vi "Change Behavior.vi"(8 "error in (no error)":errorcluster, 10 "New UI Actor":refnum<class "Flex UI (Actor).lvclass">, 11 "Flex UI (Actor) in":refnum<class "Flex UI (Actor).lvclass">) -> (0 "error out":errorcluster, 3 "Flex UI (Actor) out":refnum<class "Flex UI (Actor).lvclass">)   [LabVIEW 2014, in "Flex UI (Parent Actor).lvlib" / "Flex UI (Actor).lvclass"]
uses:
  Flex UI (Actor).lvclass
  <vilib>/East West Architects/Flex UI/Flex UI (Parent)/Flex UI.lvclass
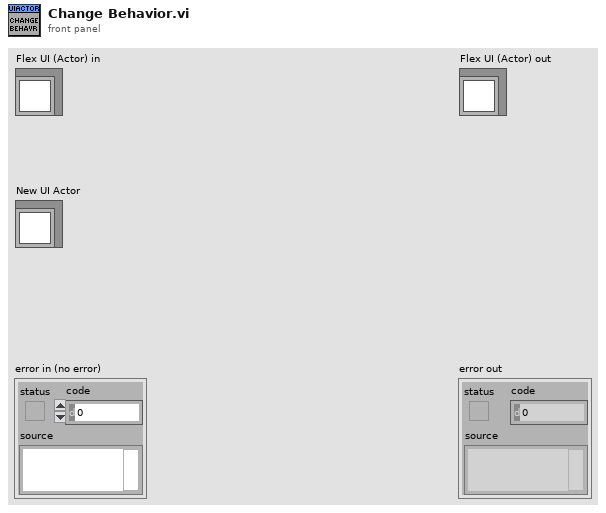
[diagram p1: front panel]
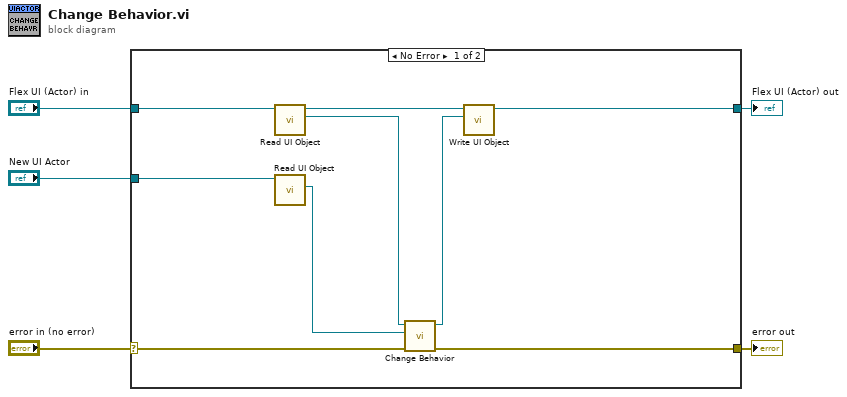
[diagram p0: block diagram]
diagram:
  n1 = case shown="No Error" "error in (no error)" {
    selector: "error in (no error)" -> [w14 w16]
    tunnel: [w13 w16] -> w4
    tunnel: [w8 w15] -> w2
    tunnel: "Flex UI (Actor) in" -> [w12 w15]
    tunnel: "New UI Actor" -> [w7 _]
    frame No Error {
      n2 = call-dynamic "Read UI Object.vi"("Flex UI (Actor) in"=w12) -> ("Flex UI Object"=w11:refnum<class "Flex UI.lvclass">, "Flex UI (Actor) out"=w10:refnum<class "Flex UI (Actor).lvclass">)  [unwired: 8 in, 1 out]
      n3 = call-dynamic "Read UI Object.vi"("Flex UI (Actor) in"=w7) -> ("Flex UI Object"=w6:refnum<class "Flex UI.lvclass">)  [unwired: 8 in, 2 out]
      n4 = call <vilib>:"Change Behavior.vi"("error in"=w14, "New Behavior"=w6, "Philips UI in"=w11) -> ("error out"=w13:errorcluster, "Philips UI out"=w9:refnum<class "Flex UI.lvclass">)  [unwired: 7 in]
      n5 = call-dynamic "Write UI Object.vi"("Flex UI in"=w9, "Flex UI (Actor) in"=w10) -> ("Flex UI (Actor) out"=w8:refnum<class "Flex UI (Actor).lvclass">)  [unwired: 8 in, 1 out]
    }
    frame Error {
    }
  }
  "error out" <- w4
  "Flex UI (Actor) out" <- w2
